vi "ReadKeyenceBoolean.vi"(9 "MemoryNumber":string, 11 "connection ID":refnum<k5>) -> (2 "status":bool, 3 "connection ID out":refnum<k5>)   [LabVIEW 2017]
panel:
  out "concatenated string":string
  out "error out":errorcluster
  out "data out":string
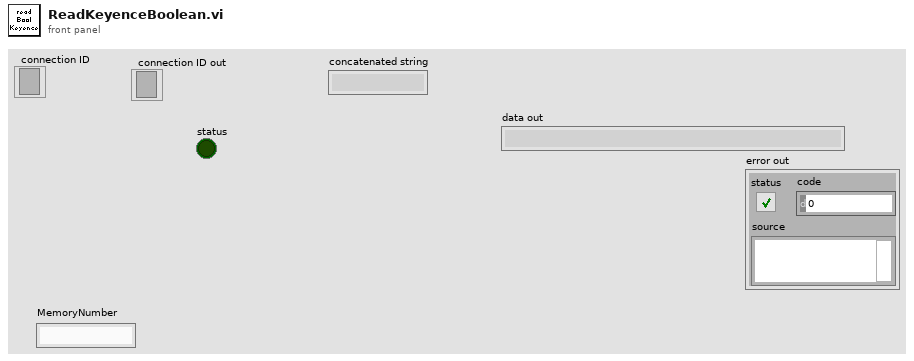
[diagram p1: front panel]
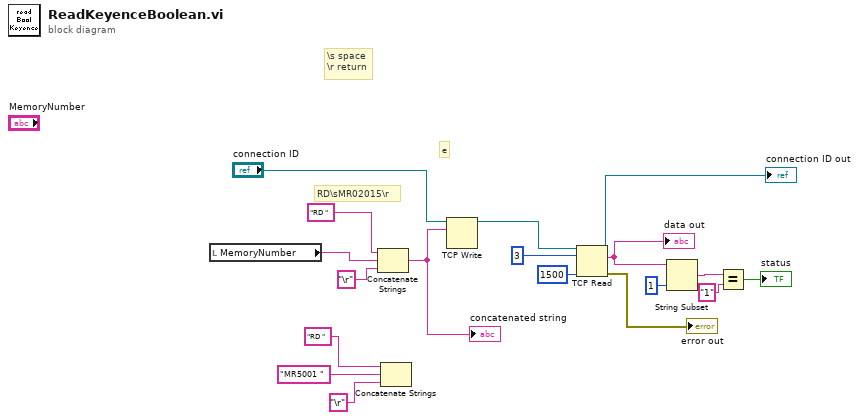
[diagram p0: block diagram]
diagram:
  # "e"
  # "\\s space\n\\r return"
  # "RD\\sMR02015\\r"
  n1 = local read "MemoryNumber"() -> (w1:string)
  n2 = Concatenate Strings("RD " ("string"), w1, "\r" ("string")) -> (w7:string)
  "concatenated string" <- w7
  n3 = Concatenate Strings("RD " ("string"), "MR5001 " ("string"), "\r" ("string")) -> ()  [unwired: 1 out]
  n4 = TCP Write(connection ID="connection ID", data in=w7) -> (connection ID out=w17:refnum<k5>)  [unwired: 2 in, 2 out]
  n5 = TCP Read(connection ID=w17, bytes to read=3, 9:1500 ("timeout ms (25000)")) -> (connection ID out=→"connection ID out":refnum<k5>, data out=w12:string, error out=→"error out":errorcluster)  [unwired: 2 in]
  "data out" <- w12
  n6 = String Subset(string=w12, length (rest)=1 ("length (rest)")) -> (substring=w10:string)  [unwired: 1 in]
  n7 = Equal?(x=w10, y="1") -> (x = y?=→"status":bool)
